vi "windowsfont.vi"(0 "x":i32, 1 "fontstyle":i32, 2 "szFaceName":string, 5 "y":i32, 7 "fontheight":i32, 9 "rotation":i32, 11 "error in (no error)":errorcluster caption="entrée d'erreur (pas d'erreur)", 12 "fontunderline":i32, 13 "content":string) -> (4 "szFaceName out":string, 6 "content out":string, 8 "function return":i32, 15 "error out":errorcluster caption="sortie d'erreur")   [LabVIEW 2020, in "Library Instrument & Equipement.lvlib" / "Library Printer.lvlib" / "TSCLIB.lvlib"]
doc: "EXPORT int CALLBACK windowsfont(int x, int y, int fontheight, int rotation, int fontstyle, int fontunderline, unsigned char *szFaceName, unsigned char *content);"
uses:
  TSCLIB.lvlib
  TSCLIB.dll
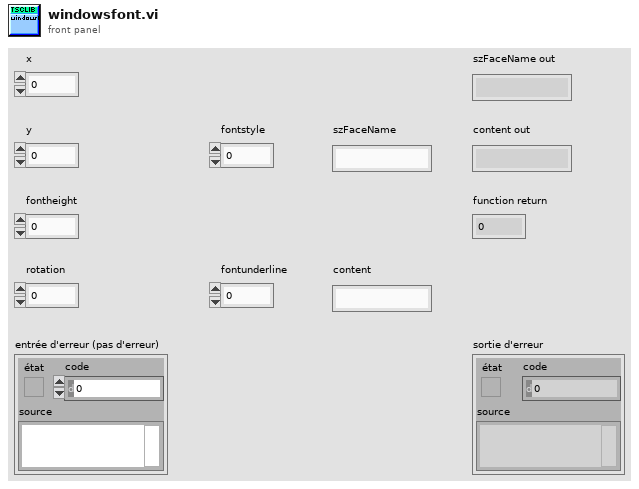
[diagram p1: front panel]
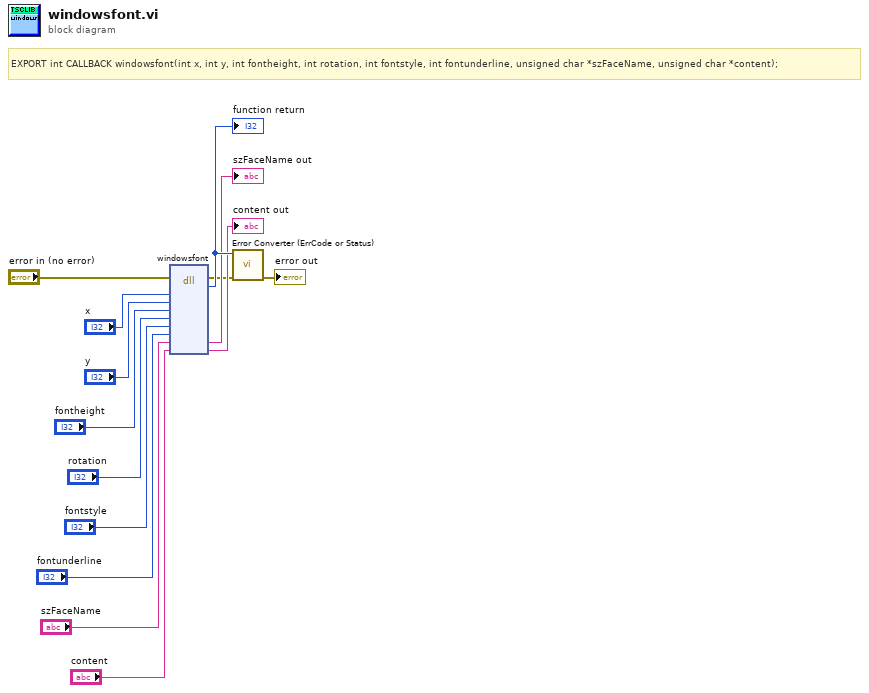
[diagram p0: block diagram]
diagram:
  # "EXPORT int CALLBACK windowsfont(int x, int y, int fontheight, int rotation, int fontstyle, int fontunderline, unsigned char *szFaceName, unsigned char *content);"
  n1 = dll-call lib="C:/Users/ngarcin/OneDrive - Altyor/Standard TB/Class/Printer/Printer TSC/TSCLIB/TSCLIB.*" fn="windowsfont"(error in="error in (no error)", "x"="x", "y"="y", "fontheight"="fontheight", "rotation"="rotation", "fontstyle"="fontstyle", "fontunderline"="fontunderline", "szFaceName"="szFaceName", "content"="content") -> (error out=w2:errorcluster, "type de retour"=w14:i32, "szFaceName"=→"szFaceName out":string, "content"=→"content out":string)  [unwired: 8 in, 1 out]
  "function return" <- w14
  n2 = call "Error Converter (ErrCode or Status).vi"("error in (no error)"=w2, "error code"=w14) -> ("error out"=→"error out":errorcluster)  [unwired: 9 in]
